vi "Polling.vi"() -> ()   [LabVIEW 2020]
doc: "Use this template to create an application that executes repeatedly until you click the Stop button. This template polls the state of the Stop button and does not use events. Use the Top-Level Application template (not available in the Base package) to create a single-loop application with event handling."
panel:
  out "error out":errorcluster
  in  "error in":errorcluster
  in  "stop":bool
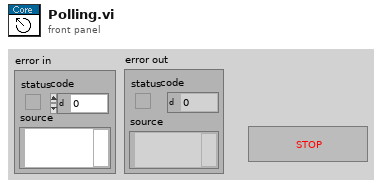
[diagram p1: front panel]
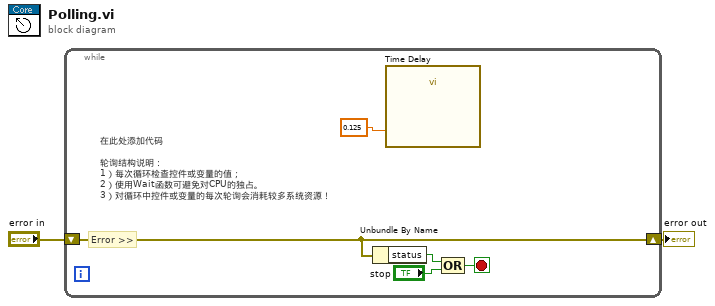
[diagram p0: block diagram]
diagram:
  n1 = while {
    shift-right: [w7] -> w1
    shift-left: "error in" -> [w7]
    stop <- w3 stop-if-true
    # "Error >>"
    # "在此处添加代码\n\n轮询结构说明：\n1）每次循环检查控件或变量的值；\n2）使用Wait函数可避免对CPU的独占。\n3）对循环中控件或变量的每次轮询会消耗较多系统资源！"
    n2 = Unbundle By Name(w7) -> ("status"=w5:bool)
    n3 = call "Time Delay"("Delay Time (s)"=0.125) -> ()  [unwired: 10 in, 1 out]
    n4 = Compound Arithmetic op=OR(w5, "stop") -> (w3:bool)
  }
  "error out" <- w1
